vi "FestoCPX.Valve(3out3in).vi"(4 "Delay [ms] (0)":u32, 6 "Timeout [ms] (5000)":u32=5000, 7 "Mode":bool, 8 "error in (no error)":errorcluster, 9 "Pos":i32, 10 "Valve outputs":T1[](array[typedef]), 11 "Inputs":T2[](array[typedef])) -> (0 "error out":errorcluster, 2 "Aborted?":bool, 3 "Timeout?":bool)   [LabVIEW 2016]
uses:
  FestoCPX.DI.Signal.ctl
  FestoCPX.DO.Signal.ctl
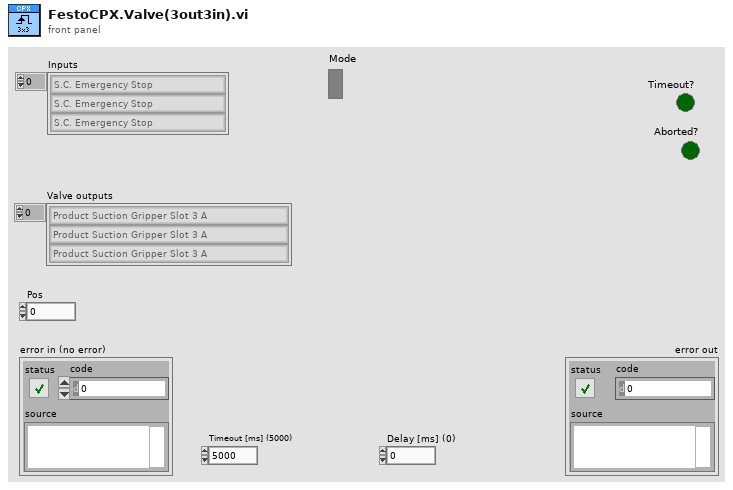
[diagram p1: front panel]
types:
  T1 = typedef "FestoCPX.DO.Signal.ctl" = enum16{"Safety Reset", "Air Main Valve", "Door Lock", "Button LED Start", "Button LED Stop", "Button LED Control", "Traffic LED Red", "Traffic LED Orange", "Traffic LED Green", "Horn", "Laser Interlock", "Laser Trigger", "Laser Fume Extractor", "Product Suction Gripper Slot 1 A", "Product Suction Gripper Slot 1 B", "Product Suction Gripper Slot 2 A", "Product Suction Gripper Slot 2 B", "Product Suction Gripper Slot 3 A", "Product Suction Gripper Slot 3 B", "Product Suction Gripper Slot 4 A", "Product Suction Gripper Slot 4 B", "Product Suction Gripper Final A", "Product Suction Gripper Final B", "Lamp", "Q1 Product Move Work", "Q1 Product Move Home", "Q2 Table Turn Work", "Q2 Table Turn Home", "Q3 Product Lift A", "Q3 Product Lift B", "Q4 Product Arm OK", "Q4 Product Arm NOK", "Q5 Product Arm Work", "Q6 Product BlowOut A", "Q6 Product BlowOut B"}
  T2 = typedef "FestoCPX.DI.Signal.ctl" = enum16{"S.C. Emergency Stop", "S.C. Side Door Close", "S.C. Front Door Close", "S.C. Front Door Secured", "Button Start", "Button Stop", "Button Control", "Product Move Home", "Product Move Work", "Table Position", "Table Lock", "Product Lift A Home", "Product Lift B Home", "Product Arm OK", "Product Arm NOK", "Product Arm Work", "Revolver ID 1", "Revolver ID 2", "Revolver ID 3", "Revolver ID 4", "Revolver ID 5", "Air Pressure Inside", "Air Pressure Inlet", "Product Slot 1 A Present", "Product Slot 1 B Present", "Product Slot 2 A Present", "Product Slot 2 B Present", "Product Slot 3 A Present", "Product Slot 3 B Present", "Product Slot 4 A Present", "Product Slot 4 B Present", "Product Final A Present", "Product Final B Present", "Product Output A Present", "Product Output B Present", "Product Container OK Present", "Product Container NOK Present", "Fork ID 1", "Fork ID 2"}
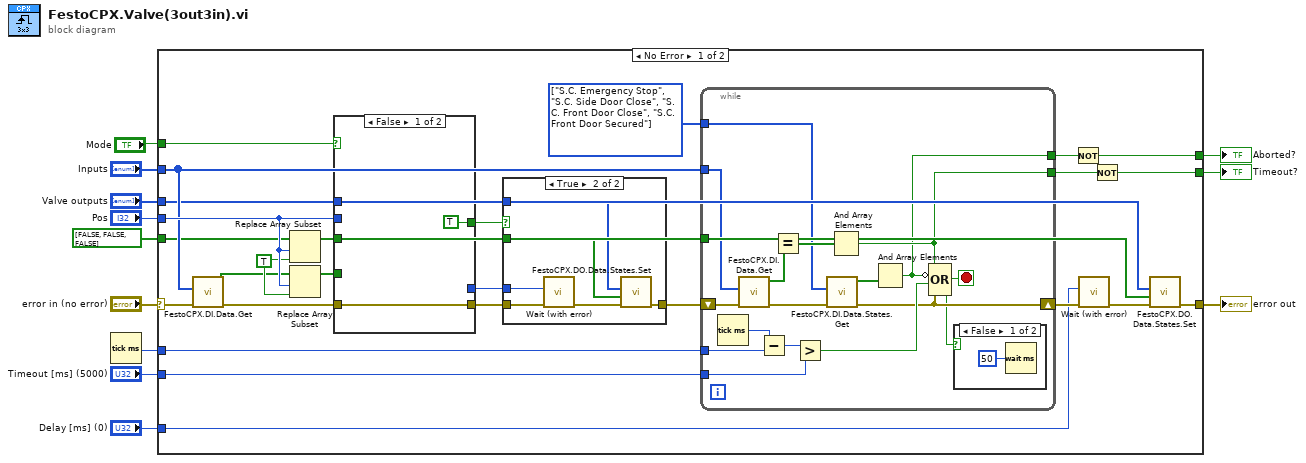
[diagram p0: block diagram]
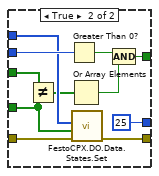
[diagram p2: hidden frame]
diagram:
  n1 = Tick Count (ms)() -> (millisecond timer value=w8:u32)
  n2 = case shown="No Error" "error in (no error)" {
    selector: "error in (no error)" -> [w26 w76]
    tunnel: "Pos" -> [w27 _]
    tunnel: [w22 w76] -> w11
    tunnel: [w35 _] -> w10
    tunnel: w8 -> [w37 _]
    tunnel: "Timeout [ms] (5000)" -> [w36 _]
    tunnel: "Inputs" -> [w24 _]
    tunnel: "Valve outputs" -> [w21 _]
    tunnel: "Delay [ms] (0)" -> [w32 _]
    tunnel: [w28 _] -> w3
    tunnel: bool[] [FALSE, FALSE, FALSE] -> [w23 _]
    tunnel: "Mode" -> [w14 _]
    frame No Error {
      w18 = TRUE ("new element/subarray")
      w30 = T2[] [enum."S.C. Emergency Stop", enum."S.C. Side Door Close", enum."S.C. Front Door Close", enum."S.C. Front Door Secured"] items=["S.C. Emergency Stop", "S.C. Side Door Close", "S.C. Front Door Close", "S.C. Front Door Secured", "Button Start", "Button Stop", "Button Control", "Product Move Home", "Product Move Work", "Table Position", "Table Lock", "Product Lift A Home", "Product Lift B Home", "Product Arm OK", "Product Arm NOK", "Product Arm Work", "Revolver ID 1", "Revolver ID 2", "Revolver ID 3", "Revolver ID 4", "Revolver ID 5", "Air Pressure Inside", "Air Pressure Inlet", "Product Slot 1 A Present", "Product Slot 1 B Present", "Product Slot 2 A Present", "Product Slot 2 B Present", "Product Slot 3 A Present", "Product Slot 3 B Present", "Product Slot 4 A Present", "Product Slot 4 B Present", "Product Final A Present", "Product Final B Present", "Product Output A Present", "Product Output B Present", "Product Container OK Present", "Product Container NOK Present", "Fork ID 1", "Fork ID 2"] ("CPX.DI")
      n3 = call-poly "FestoCPX.DI.Data.Get.vi"("error in (no error)"=w26, "CPX.DI"=w24) -> ("error out"=w25:errorcluster, "State"=w15:bool[])  [unwired: 5 in, 3 out]
      n4 = Replace Array Subset(array=w23, new element=w18, index=w27) -> (w16:bool[])
      n5 = Replace Array Subset(array=w15, new element=w18, index=w27) -> (w19:bool[])
      n6 = case shown="False" w14 {
        tunnel: w27 -> [_ w50]
        tunnel: w25 -> [w39 w49]
        tunnel: w21 -> [_ w48]
        tunnel: [w39 w47] -> w20
        tunnel: w19 -> [_ w46]
        tunnel: [TRUE w45] -> w17
        tunnel: w16 -> [_ w44]
        tunnel: [_ u32 25 ("milliseconds to wait")] -> w13
        frame False {
        }
        frame True {
          n7 = Not Equal?(x=w44, y=w46) -> (x != y?=w43:bool[])
          n8 = Greater Than 0?(x=w50) -> (x > 0?=w41:bool)
          n9 = Or Array Elements(Boolean array=w43) -> (logical OR=w42:bool)
          n10 = call "FestoCPX.DO.Data.States.Set.vi"("error in (no error)"=w49, "State"=w46, "CPX.DO"=w48) -> ("error out"=w47:errorcluster)  [unwired: 8 in]
          n11 = Compound Arithmetic op=AND(w41, w42) -> (w45:bool)
        }
      }
      n12 = case shown="True" w17 {
        tunnel: [w51 w57] -> w31
        tunnel: w21 -> [_ w56]
        tunnel: w20 -> [w51 w55]
        tunnel: w16 -> [_ w53]
        tunnel: w13 -> [_ w52]
        frame False {
        }
        frame True {
          n13 = call "Wait (with error).vi"("error in (no error)"=w55, "milliseconds to wait"=w52) -> ("error out"=w54:errorcluster)  [unwired: 8 in, 1 out]
          n14 = call "FestoCPX.DO.Data.States.Set.vi"("error in (no error)"=w54, "State"=w53, "CPX.DO"=w56) -> ("error out"=w57:errorcluster)  [unwired: 8 in]
        }
      }
      n15 = while {
        shift-right: [w63] -> w33
        shift-left: w31 -> [w74]
        tunnel: w24 -> [w73]
        tunnel: [w66] -> w34
        tunnel: w37 -> [w71]
        tunnel: w36 -> [w69]
        tunnel: w16 -> [w68]
        tunnel: w30 -> [w62]
        tunnel: [w61] -> w29
        stop <- w60 stop-if-true
        n16 = Tick Count (ms)() -> (millisecond timer value=w72:u32)
        n17 = call-poly "FestoCPX.DI.Data.Get.vi"("error in (no error)"=w74, "CPX.DI"=w73) -> ("error out"=w64:errorcluster, "State"=w59:bool[])  [unwired: 5 in, 3 out]
        n18 = Subtract(x=w72, y=w71) -> (x-y=w70:u32)
        n19 = Equal?(x=w68, y=w59) -> (x = y?=w67:bool[])
        n20 = Greater?(x=w70, y=w69) -> (0:w65:bool)
        n21 = call "FestoCPX.DI.Data.States.Get.vi"("error in (no error)"=w64, "CPX.DI"=w62) -> ("error out"=w63:errorcluster, "State"=w58:bool[])  [unwired: 5 in, 3 out]
        n22 = And Array Elements(Boolean array=w67) -> (logical AND=w66:bool)
        n23 = And Array Elements(Boolean array=w58) -> (logical AND=w61:bool)
        n24 = Compound Arithmetic op=OR(w66, invert w61, w65, w63) -> (w60:bool)
        n25 = case shown="False" w60 {
          frame False {
            n26 = Wait (ms)(milliseconds to wait=u32 50) -> ()  [unwired: 1 out]
          }
          frame True {
          }
        }
      }
      n27 = Not(x=w29) -> (.not. x?=w28:bool)
      n28 = call "Wait (with error).vi"("error in (no error)"=w33, "milliseconds to wait"=w32) -> ("error out"=w22:errorcluster)  [unwired: 8 in, 1 out]
      n29 = Not(x=w34) -> (.not. x?=w35:bool)
      n30 = call "FestoCPX.DO.Data.States.Set.vi"("error in (no error)"=w22, "State"=w16, "CPX.DO"=w21) -> ()  [unwired: 8 in, 1 out]
    }
    frame Error {
    }
  }
  "error out" <- w11
  "Timeout?" <- w10
  "Aborted?" <- w3
